vi "AutoRoutineSelector.vi"(4 "NotPurePursuit":bool, 5 "OurSwitch":bool, 6 "RR":dbl, 7 "OurScale":bool, 8 "RL":dbl, 9 "LR":dbl, 10 "LL":dbl, 11 "Position":dbl) -> (3 "File Name":string)   [LabVIEW 2017]
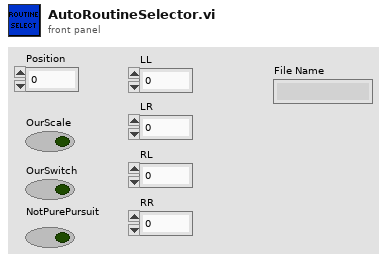
[diagram p1: front panel]
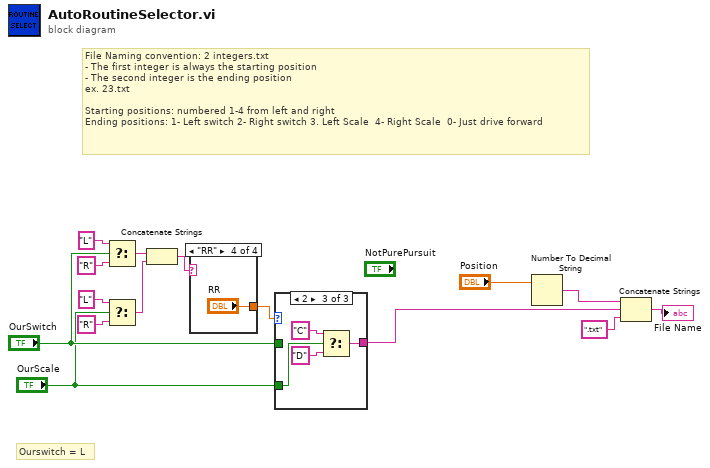
[diagram p0: block diagram]
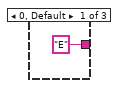
[diagram p2: hidden frame]
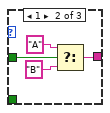
[diagram p3: hidden frame]
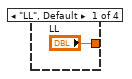
[diagram p4: hidden frame]
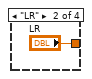
[diagram p5: hidden frame]
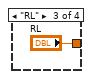
[diagram p6: hidden frame]
diagram:
  # "Ourswitch = L"
  # "File Naming convention: 2 integers.txt \n- The first integer is always the starting position\n- The second integer is the ending position\nex. 23.txt\n\nStarting positions: numbered 1-4 from left and right\nEnding positions: 1- Left switch 2- Right switch 3. Left Scale  4- Right Scale  0- Just drive forward"
  n1 = Select(t="L", s="OurSwitch", f="R") -> (s? t:f=w10:string)
  n2 = Select(t="L", s="OurScale", f="R") -> (s? t:f=w9:string)
  n3 = Concatenate Strings(w10, w9) -> (w8:string)
  n4 = case shown="\"RR\"" w8 {
    tunnel: ["LL" "LR" "RL" "RR"] -> w7
    frame "LL", Default {
    }
    frame "LR" {
    }
    frame "RL" {
    }
    frame "RR" {
    }
  }
  n5 = case shown="2" w7 {
    tunnel: "OurSwitch" -> [_ w22 _]
    tunnel: "OurScale" -> [_ _ w26]
    tunnel: ["E" w21 w25] -> w2
    frame 0, Default {
    }
    frame 1 {
      n6 = Select(t="A", s=w22, f="B") -> (s? t:f=w21:string)
    }
    frame 2 {
      n7 = Select(t="C", s=w26, f="D") -> (s? t:f=w25:string)
    }
  }
  n8 = Number To Decimal String(number="Position") -> (decimal integer string=w3:string)  [unwired: 1 in]
  n9 = Concatenate Strings(w3, w2, ".txt") -> (→"File Name":string)
